vi "get pixel clock.vi"(8 "error in (no error)":errorcluster, 11 "Thorcam in":refnum<class "Thorcam.lvclass">) -> (0 "error out":errorcluster, 3 "Thorcam out":refnum<class "Thorcam.lvclass">)   [LabVIEW 2012, in "Thorcam.lvclass"]
uses:
  Thorcam.lvclass
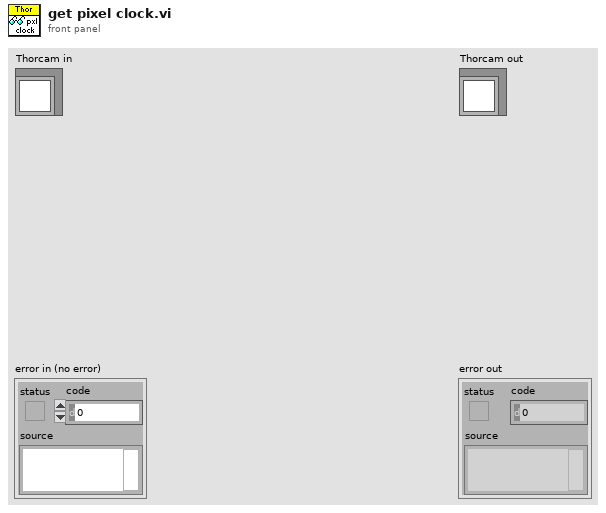
[diagram p1: front panel]
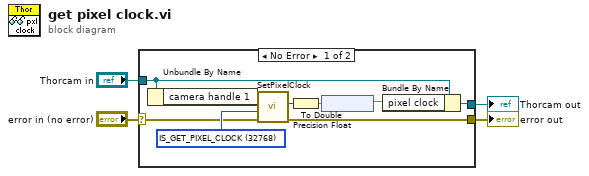
[diagram p0: block diagram]
diagram:
  n1 = case shown="No Error" "error in (no error)" {
    selector: "error in (no error)" -> [w10 w15]
    tunnel: [w9 w15] -> w3
    tunnel: [w7 w14] -> w1
    tunnel: "Thorcam in" -> [w8 w14]
    frame No Error {
      w11 = 32768 items=["IS_GET_PIXEL_CLOCK"=32768, "IS_GET_DEFAULT_PCLK"=32769, "IS_SET_PIXEL_CLOCK"=32770] ("Mode")
      n2 = Unbundle By Name(w8) -> ("camera handle 1"=w5:u32)
      n3 = call <instrlib>:"SetPixelClock.vi"("error in"=w10, "Mode"=w11, "Camera Handle In"=w5) -> ("error out"=w9:errorcluster, "Value"=w12:i32)  [unwired: 6 in, 1 out]
      n4 = To Double Precision Float(number=w12) -> (double precision float=w13:dbl)
      n5 = node(w13) -> (w6:dbl[unit])
      n6 = Bundle By Name(cluster=w8, "pixel clock"=w6) -> (w7:refnum<class "Thorcam.lvclass">)
    }
    frame Error {
    }
  }
  "error out" <- w3
  "Thorcam out" <- w1
